vi "Subset.vi"(8 "error in (no error)":errorcluster, 9 "Count":i32, 10 "Start":i32, 11 "TermBuffer in":refnum<class "TermBuffer.lvclass">) -> (0 "error out":errorcluster, 2 "Lines":refnum<class "TermLine.lvclass">[](array[class]), 3 "TermBuffer out":refnum<class "TermBuffer.lvclass">)   [LabVIEW 2020, in "Terminal.lvlib" / "TermBuffer.lvclass"]
uses:
  TermBuffer.lvclass
  TermBuffer.lvclass/TermBuffer.ctl
  TermLine/TermLine.lvclass
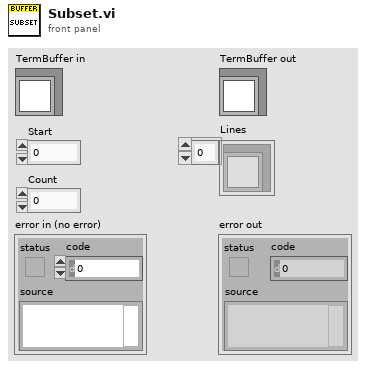
[diagram p1: front panel]
types:
  T1 = typedef "Terminal.lvlib/TermBuffer.lvclass/Ref Data.ctl" = cluster{"Lines":refnum<class "TermLine.lvclass">[], "Rows":i32, "Cols":i32}
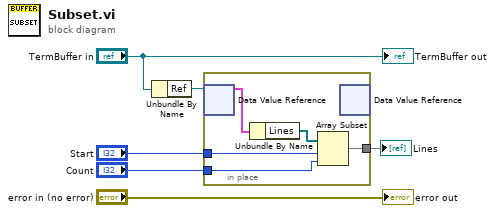
[diagram p0: block diagram]
diagram:
  n1 = Unbundle By Name("TermBuffer in") -> ("Ref"=w5:refnum<data-value>)
  n2 = in-place {
    in-place-border: [w9] -> w3
    in-place-border: "Start" -> [w8]
    in-place-border: "Count" -> [w7]
    n3 = in-place-dvr #1(w5) -> (w11:T1)  [unwired: 1 out]
    n4 = Unbundle By Name(w11) -> ("Lines"=w10:refnum<class "TermLine.lvclass">[])
    n5 = Array Subset(array=w10, index=w8, length=w7) -> (w9:refnum<class "TermLine.lvclass">[])
    n6 = in-place-dvr #1() -> ()  [unwired: 1 in, 2 out]
  }
  "Lines" <- w3
  "error out" <- "error in (no error)"
  "TermBuffer out" <- "TermBuffer in"
